vi "colornn.vi"(5 "error in":errorcluster) -> (0 "green":i32, 1 "yellow":i32, 14 "black":i32, 15 "blue":i32, 16 "red":i32, 19 "error out":errorcluster)   [LabVIEW 2019]
panel:
  out "Image Out":T1(plugin-control)
  in  "Stop (F)":bool
  out "Matches (calibrated) (green)":T2(array[cluster]) {"Bounding Box"."y" format="%.2f"; "Bounding Box"."x" format="%.2f"; "Position"."y" format="%.2f"; "Position"."x" format="%.2f"; "Score" format="%.2f"; "Scale" format="%.2f"; "Angle" format="%.2f"}
  out "Matches (calibrated) (yellow)":T2(array[cluster]) {"Bounding Box"."y" format="%.2f"; "Bounding Box"."x" format="%.2f"; "Position"."y" format="%.2f"; "Position"."x" format="%.2f"; "Score" format="%.2f"; "Scale" format="%.2f"; "Angle" format="%.2f"}
  out "Matches (calibrated) (black)":T2(array[cluster]) {"Bounding Box"."y" format="%.2f"; "Bounding Box"."x" format="%.2f"; "Position"."y" format="%.2f"; "Position"."x" format="%.2f"; "Score" format="%.2f"; "Scale" format="%.2f"; "Angle" format="%.2f"}
  out "Matches (calibrated) (red)":T2(array[cluster]) {"Bounding Box"."y" format="%.2f"; "Bounding Box"."x" format="%.2f"; "Position"."y" format="%.2f"; "Position"."x" format="%.2f"; "Score" format="%.2f"; "Scale" format="%.2f"; "Angle" format="%.2f"}
  out "Matches (calibrated) (blue)":T2(array[cluster]) {"Bounding Box"."y" format="%.2f"; "Bounding Box"."x" format="%.2f"; "Position"."y" format="%.2f"; "Position"."x" format="%.2f"; "Score" format="%.2f"; "Scale" format="%.2f"; "Angle" format="%.2f"}
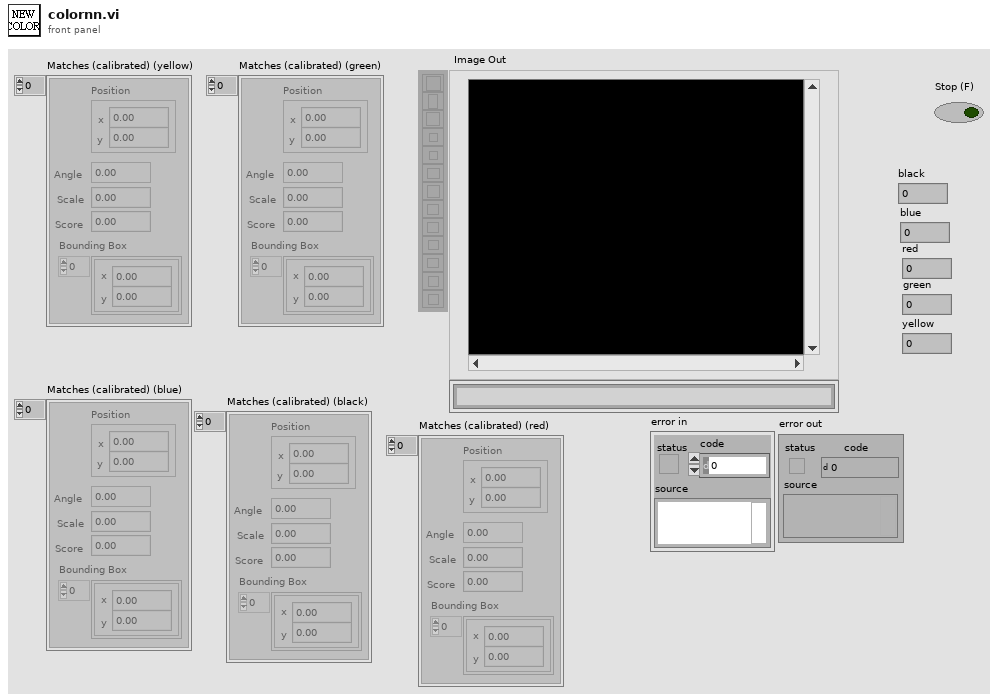
[diagram p1: front panel]
types:
  T1 = typedef "IMAQ Image.ctl" = refnum<image>
  T2 = cluster{"Position":cluster{"x":sgl, "y":sgl}, "Angle":sgl, "Scale":sgl, "Score":sgl, "Bounding Box":cluster{"x":sgl, "y":sgl}[]}[]
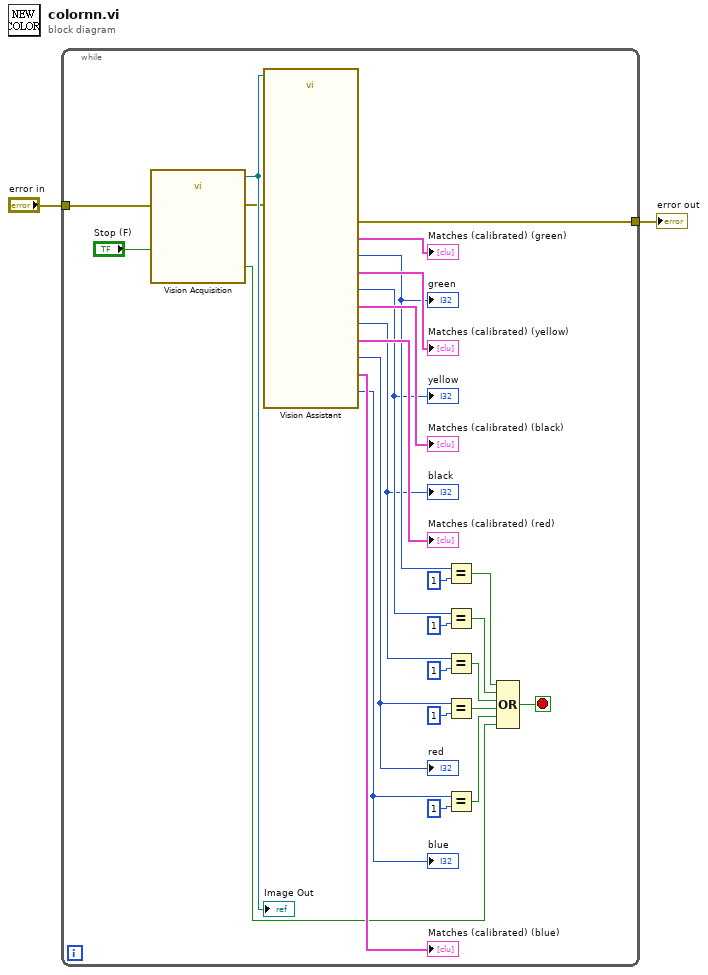
[diagram p0: block diagram]
diagram:
  n1 = while {
    tunnel: [w5] -> w2
    tunnel: "error in" -> [w4]
    stop <- w6 stop-if-true
    n2 = call "Vision Acquisition"("Stop (F)"="Stop (F)", "error in"=w4) -> ("Image Out"=w28:T1, "Stopped"=w7:bool, "error out"=w3:errorcluster)  [unwired: 23 in]
    "Image Out" <- w28
    n3 = call "Vision Assistant"("Image In"=w28, "error in"=w3) -> ("Number of Matches (blue)"=w13:i32, "Matches (calibrated) (blue)"=→"Matches (calibrated) (blue)":T2, "Number of Matches (red)"=w15:i32, "Matches (calibrated) (red)"=→"Matches (calibrated) (red)":T2, "Matches (calibrated) (green)"=→"Matches (calibrated) (green)":T2, "Number of Matches (green)"=w22:i32, "Matches (calibrated) (yellow)"=→"Matches (calibrated) (yellow)":T2, "Number of Matches (yellow)"=w19:i32, "Matches (calibrated) (black)"=→"Matches (calibrated) (black)":T2, "Number of Matches (black)"=w17:i32, "error out"=w5:errorcluster)  [unwired: 14 in, 1 out]
    "green" <- w22
    "yellow" <- w19
    "black" <- w17
    "red" <- w15
    "blue" <- w13
    n4 = Equal?(x=w22, y=1) -> (x = y?=w12:bool)
    n5 = Equal?(x=w19, y=1) -> (x = y?=w11:bool)
    n6 = Equal?(x=w17, y=1) -> (x = y?=w10:bool)
    n7 = Equal?(x=w15, y=1) -> (x = y?=w9:bool)
    n8 = Equal?(x=w13, y=1) -> (x = y?=w8:bool)
    n9 = Compound Arithmetic op=OR(w12, w11, w10, w9, w8, w7) -> (w6:bool)
  }
  "error out" <- w2
